vi "Init.vi"(8 "error in":errorcluster, 11 "IData Sink in":refnum<class "IData Sink.lvclass">) -> (0 "error out":errorcluster, 3 "IData Sink out":refnum<class "IData Sink.lvclass">)   [LabVIEW 2024, in "IData Sink.lvclass"]
uses:
  IData Sink.lvclass
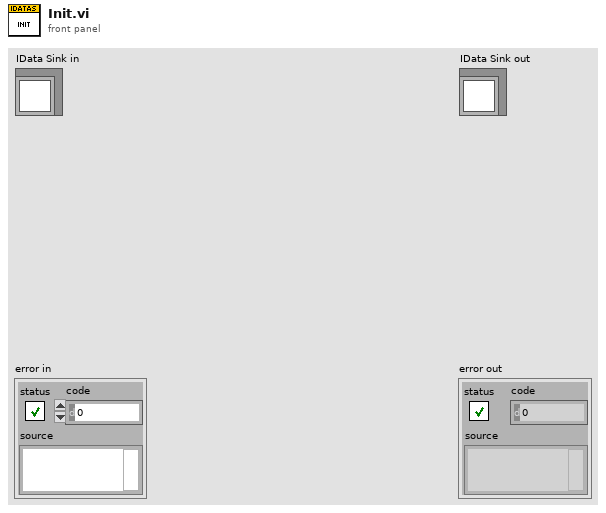
[diagram p1: front panel]
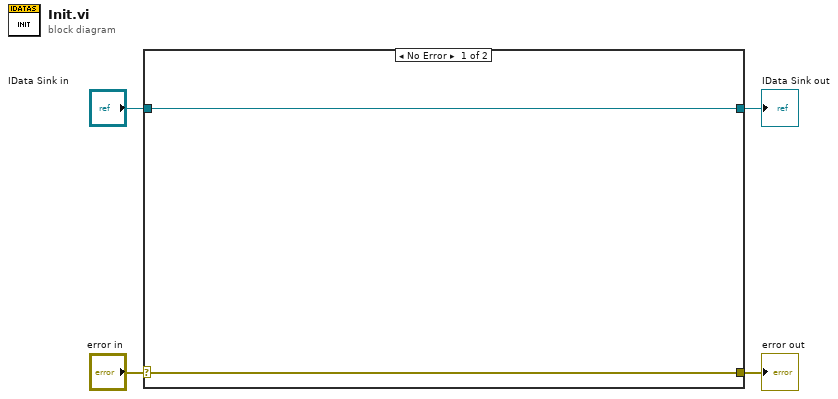
[diagram p0: block diagram]
diagram:
  n1 = case shown="No Error" "error in" {
    selector: "error in" -> [w5 w8]
    tunnel: [w5 w8] -> w3
    tunnel: [w6 w7] -> w1
    tunnel: "IData Sink in" -> [w6 w7]
    frame No Error {
    }
    frame Error {
    }
  }
  "error out" <- w3
  "IData Sink out" <- w1
